vi "创建模板.vi"(2 "模板图片名":string, 3 "源图片":T1) -> (1 "模板":T1(plugin-control))   [LabVIEW 2014]
uses:
  <vilib>/vision/Image Controls.llb/IMAQ Image.ctl
  <vilib>/vision/NI_Vision_Development_Module.lvlib
panel:
  # "从源图片中截取模板，并生成模板的信息报告"
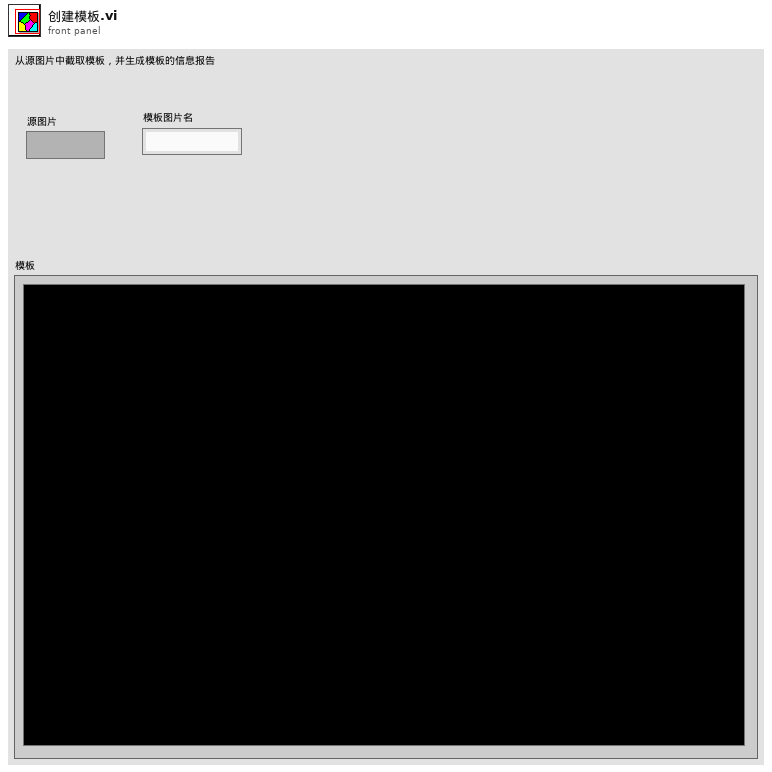
[diagram p1: front panel]
types:
  T1 = typedef "IMAQ Image.ctl" = refnum<image>
  T2 = typedef "Image Type" = u32
  T3 = typedef "ROI Descriptor" = cluster{"Global Rectangle":i32[], "Contours":cluster{"ID":enum32{"External", "Internal"}, "Type":u32, "Coordinates":i32[]}[]}
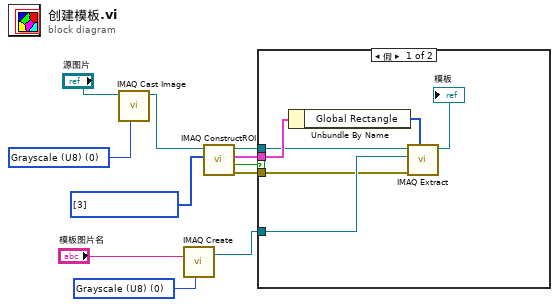
[diagram p0: block diagram]
diagram:
  w3 = T2 0 items=["Grayscale (U8)", "Grayscale (I16)", "Grayscale (SGL)", "Complex (CSG)", "RGB (U32)", "HSL (U32)", "RGB (U64)", "Grayscale (U16)"] ("Image Type")
  w5 = T2 0 items=["Grayscale (U8)", "Grayscale (I16)", "Grayscale (SGL)", "Complex (CSG)", "RGB (U32)", "HSL (U32)", "RGB (U64)", "Grayscale (U16)"] ("Image Type")
  w11 = u32[] [3] items=["No Selection", "Point", "Line", "Rectangle", "Oval", "Polygon", "Freehand Region", "Annulus", "Zoom", "Pan", "Broken Line", "Freehand Line", "Rotated Rectangle"] ("Tools")
  n1 = call "IMAQ Cast Image"("Image Type"=w3, "Image Src"="源图片") -> ("Image Dst Out"=w1:T1)  [unwired: 8 in, 1 out]
  n2 = call "IMAQ Create"("Image Name"="模板图片名", "Image Type"=w5) -> ("New Image"=w6:T1)  [unwired: 3 in, 1 out]
  n3 = call "IMAQ ConstructROI"("Tools"=w11, "Image"=w1) -> ("error out"=w7:errorcluster, "Cancel"=w10:bool, "ROI Descriptor Out"=w8:T3, "Image Out (duplicate)"=w9:T1)  [unwired: 6 in]
  n4 = case shown="假" w10 {
    tunnel: w9 -> [w15 _]
    tunnel: w8 -> [w16 _]
    tunnel: w6 -> [w14 _]
    tunnel: w7 -> [w13 _]
    frame False {
      n5 = Unbundle By Name(w16) -> ("Global Rectangle"=w17:i32[])
      n6 = call "IMAQ Extract"("Optional Rectangle"=w17, "error in (no error)"=w13, "Image Dst"=w14, "Image Src"=w15) -> ("Image Dst Out"=→"模板":T1)  [unwired: 6 in, 1 out]
    }
    frame True {
    }
  }
